vi "Get Arduino Base Path.vi"(8 "Error In":errorcluster) -> (0 "Error Out":errorcluster, 3 "Arduino Base Path":path)   [LabVIEW 2014]
uses:
  <vilib>/Utility/config.llb/Read Key (Path).vi
  <vilib>/Utility/config.llb/NI_LVConfig.lvlib
  <vilib>/MakerHub/Toolbox/LMH-Toolbox.lvlib
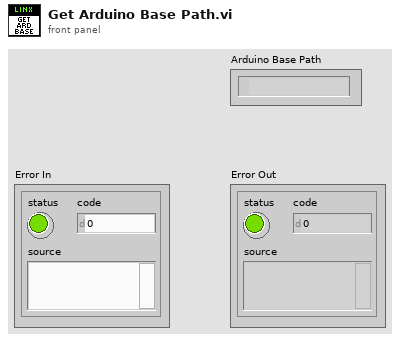
[diagram p1: front panel]
types:
  T1 = typedef "NI_LVConfig.lvlib/Config Data RefNum.ctl" = refnum<k1>
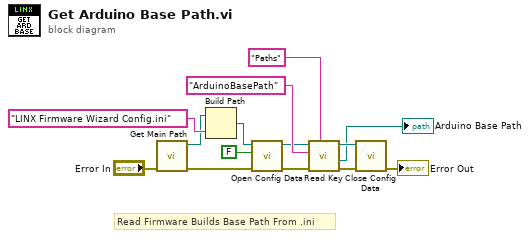
[diagram p0: block diagram]
diagram:
  # "Read Firmware Builds Base Path From .ini"
  n1 = call <vilib>:"Get Main Path.vi"("Error In"="Error In") -> ("Error Out"=w2:errorcluster, "Main Dir"=w5:path)  [unwired: 8 in, 1 out]
  n2 = Build Path(base path=w5, name or relative path="LINX Firmware Wizard Config.ini") -> (appended path=w4:path)
  n3 = call <vilib>:"Open Config Data.vi"("error in (no error)"=w2, "create file if necessary (T)"=FALSE, "configuration file path"=w4) -> ("error out"=w10:errorcluster, "refnum"=w11:T1)  [unwired: 6 in, 1 out]
  n4 = call-poly <vilib>:"Read Key.vi"("section"="Paths", "error in (no error)"=w10, "key"="ArduinoBasePath", "refnum"=w11) -> ("error out"=w9:errorcluster, "value"=→"Arduino Base Path":path, "refnum out"=w7:T1)  [unwired: 4 in, 1 out]
  n5 = call <vilib>:"Close Config Data.vi"("error in (no error)"=w9, "refnum"=w7) -> ("error out"=→"Error Out":errorcluster)  [unwired: 8 in, 1 out]
